vi "Log Event.vi"(0 "Robot Notifications in":refnum<class "Robot Event SystemLink.lvclass">, 1 "Program":string, 2 "data":variant, 5 "error in (no error)":errorcluster, 9 "Event Type":T1) -> (14 "Robot Notifications out":refnum<class "Robot Event SystemLink.lvclass">, 19 "error out":errorcluster)   [LabVIEW 2019, in "Robot Event SystemLink.lvclass"]
uses:
  Robot Event SystemLink.lvclass
  C:/_Code/Development/Sub-Zero Functional Test/standard hardware/Universal Robots/UR LabVIEW Interface/Classes/Events/Robot Event/Robot Event.lvclass
  Robot Event/Event Type.ctl
  Robot Event SystemLink.lvclass/Robot Event SystemLink.ctl
  <vilib>/Skyline/Alarm/Library/typedefs/Severity Level.ctl
  <vilib>/Skyline/Alarm/Library/typedefs/New Instance Information.ctl
  <vilib>/Skyline/Utilities/Property.ctl
  <vilib>/Skyline/Configuration/Configuration HTTP_class/NI Skyline Configuration HTTP.lvclass/NI Skyline Configuration HTTP.ctl
  <vilib>/Skyline/Notification/Class/NI SystemLink Notification.lvclass/NI SystemLink Notification.ctl
  <vilib>/Skyline/Notification/Class/Read Display Name.vi
  <vilib>/Skyline/Alarm/Class/Build Alarm Set Transition (Single Notification).vi
  <vilib>/Skyline/Configuration/Configuration HTTP_class/Read Configuration.vi
  <vilib>/Skyline/Notification/Class/Get Notification Strategies Core.vi
  <vilib>/Skyline/Notification/Class/Read ID.vi
  <vilib>/Skyline/Alarm/Class/Build Alarm Set Transition (Multiple Notifications).vi
  <vilib>/Skyline/Alarm/Class/Private/Add System to Properties.vi
  <vilib>/Skyline/Notification/Class/Initialize.vi
  <vilib>/Skyline/AssetManagement/Start Utilization (Single).vi
  <vilib>/Skyline/Utilities/Build Resource Name.vi
  <vilib>/Skyline/Utilities/Get Minion ID.vi
  <vilib>/Skyline/Utilities/Get System Name.vi
  <vilib>/Skyline/Alarm/Library/Community/Create or Update Alarm.vi
  <vilib>/Skyline/Configuration/Configuration HTTP_class/NI Skyline Configuration HTTP.lvclass
  <vilib>/Skyline/Notification/Class/NI SystemLink Notification.lvclass
  <vilib>/Skyline/Alarm/Class/NI SystemLink Alarm.lvclass
  <vilib>/Skyline/Alarm/Library/NI SystemLink Alarm Library.lvlib
  <vilib>/Skyline/Utilities/NI Skyline Utilities.lvlib
  <vilib>/Skyline/AssetManagement/NI SystemLink Asset Utilization.lvclass
  Robot Event/Robot Event.lvclass
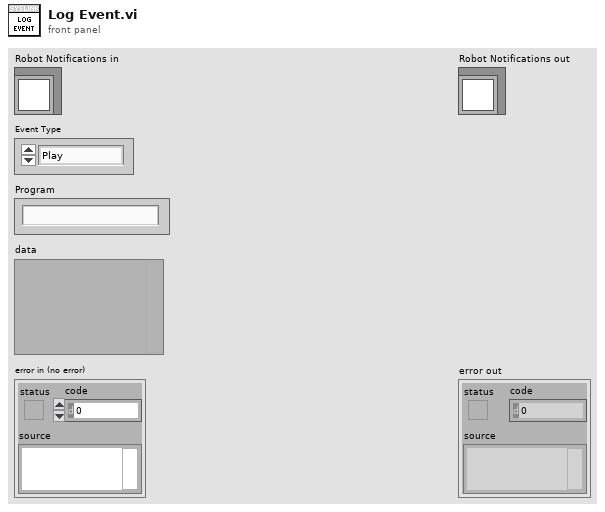
[diagram p1: front panel]
types:
  T1 = typedef "Robot Event.lvclass/Event Type.ctl" = enum16{"Play", "Error", "Fault", "Timeout", "Stopped", "Complete", "Fault - Program Resumed", "Fault - Program Aborted"}
  T2 = typedef "NI Skyline Utilities.lvlib/Property.ctl" = cluster{"key":string, "value":string}
  T3 = typedef "NI SystemLink Alarm Library.lvlib/New Instance Information.ctl" = cluster{"created by":string, "description":string, "keywords":string[], "properties":T2[]}
  T4 = typedef "NI SystemLink Alarm Library.lvlib/Severity Level.ctl" = i32
  T5 = typedef "NI SystemLink Alarm.lvclass/Set Transition.ctl" = cluster{"severity level":T4, "condition":string, "occurred at":timestamp, "notification strategies":refnum<class "NI SystemLink Notification.lvclass">[], "keywords":string[], "properties":T2[]}
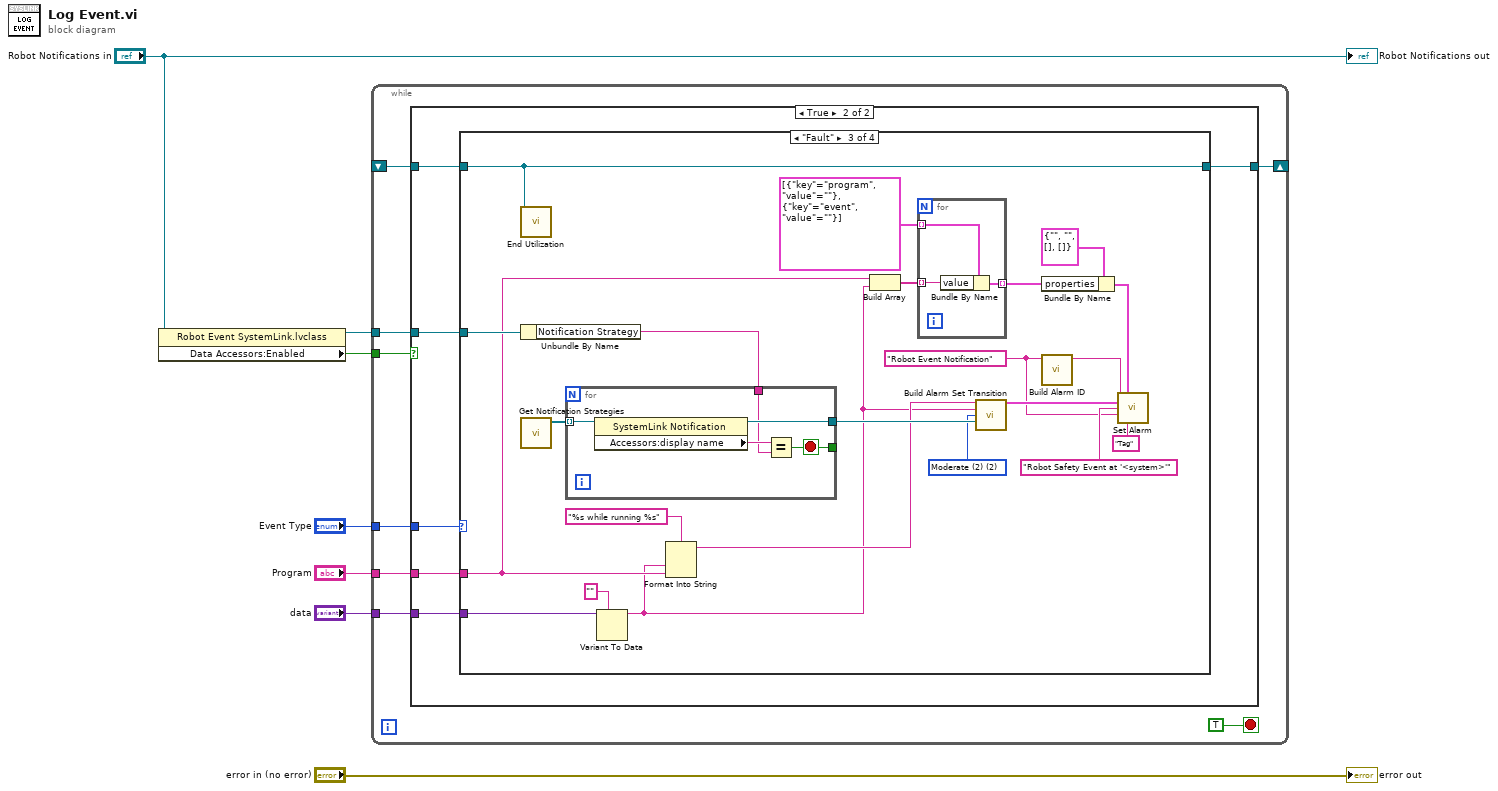
[diagram p0: block diagram]
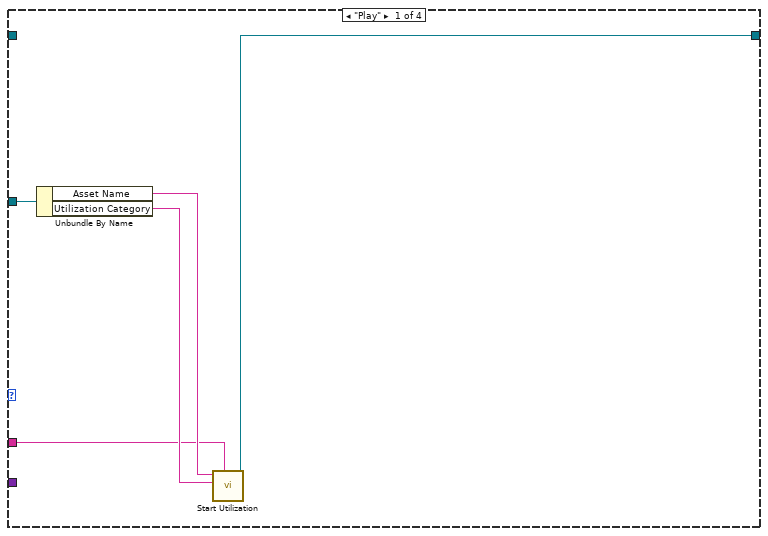
[diagram p3: hidden frame]
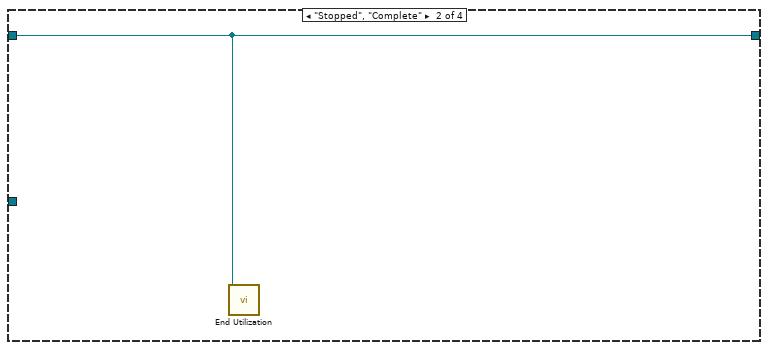
[diagram p4: hidden frame]
diagram:
  n1 = property class="Robot Event SystemLink.lvclass"(reference="Robot Notifications in") -> (reference out=w3:refnum<class "Robot Event SystemLink.lvclass">, "Data Accessors:Enabled"=w1:bool)  [unwired: 1 in, 1 out]
  n2 = while {
    tunnel: "Event Type" -> [w15]
    tunnel: "Program" -> [w14]
    tunnel: w3 -> [w13]
    tunnel: "data" -> [w12]
    tunnel: w1 -> [w11]
    shift-right: [w9] -> _
    shift-left: _ -> [w8]
    stop <- TRUE stop-if-true
    n3 = case shown="True" w11 {
      tunnel: w15 -> [_ w19]
      tunnel: w12 -> [_ w21]
      tunnel: w14 -> [_ w20]
      tunnel: w13 -> [_ w22]
      tunnel: [w16 w18] -> w9
      tunnel: w8 -> [w16 w17]
      frame False {
      }
      frame True {
        n4 = case shown="\"Fault\"" w19 {
          tunnel: w22 -> [w27 _ w50 _]
          tunnel: w21 -> [_ _ w45 _]
          tunnel: w20 -> [w23 _ w35 _]
          tunnel: [w24 w28 w29 w59] -> w18
          tunnel: w17 -> [_ w28 w29 w59]
          frame "Play" {
            n5 = Unbundle By Name(w27) -> ("Asset Name"=w26:string, "Utilization Category"=w25:string)
            n6 = call-poly <vilib>:"Start Utilization.vi"("task name"=w23, "utilization category"=w25, "asset name"=w26) -> ("asset utilization"=w24:refnum<class "NI SystemLink Asset Utilization.lvclass">)  [unwired: 7 in, 1 out]
          }
          frame "Stopped", "Complete" {
            n7 = call <vilib>:"End Utilization.vi"("asset utilization"=w28) -> ()  [unwired: 10 in, 1 out]
          }
          frame "Fault" {
            w38 = "Robot Event Notification" ("alarm name")
            w46 = T4 2 items=["Clear (-1)"=-1, "Low (1)"=1, "Moderate (2)"=2, "High (3)"=3, "Critical (4)"=4] ("severity level")
            n8 = call <vilib>:"End Utilization.vi"("asset utilization"=w29) -> ()  [unwired: 10 in, 1 out]
            n9 = Unbundle By Name(w50) -> ("Notification Strategy"=w48:string)
            n10 = call <vilib>:"Get Notification Strategies.vi"() -> ("notification strategies"=w49:refnum<class "NI SystemLink Notification.lvclass">[])  [unwired: 10 in, 1 out]
            n11 = for {
              tunnel: w49 -> [w58] mode=indexing
              tunnel: [w57] -> w47
              tunnel: w48 -> [w55]
              tunnel: [w54] -> _
              stop <- w54 stop-if-true
              n12 = property class="SystemLink Notification"(reference=w58) -> (reference out=w57:refnum<class "NI SystemLink Notification.lvclass">, "Accessors:display name"=w56:string)  [unwired: 1 in, 1 out]
              n13 = Equal?(x=w56, y=w55) -> (x = y?=w54:bool)
            }
            n14 = Variant To Data(type="", Variant=w45) -> (data=w34:string)  [unwired: 1 in, 1 out]
            n15 = Format Into String(format string="%s while running %s", w34, w35) -> (resulting string=w42:string)  [unwired: 2 in, 1 out]
            n16 = Build Array(w35, w34) -> (w33:string[])
            n17 = for {
              tunnel: w33 -> [w53] mode=indexing
              tunnel: [w52] -> w31 mode=indexing
              tunnel: T2[] [{"key"="program", "value"=""}, {"key"="event", "value"=""}] ("properties") -> [w51] mode=indexing
              n18 = Bundle By Name(cluster=w51, "value"=w53) -> (w52:T2)
            }
            n19 = call-poly <vilib>:"Build Alarm Set Transition.vi"("value"=w42, "condition"=w34, "severity level"=w46, "notification strategy"=w47) -> ("set transition"=w41:T5)  [unwired: 11 in]
            n20 = Bundle By Name(cluster=T3 {"created by"="", "description"="", "keywords"=[], "properties"=[]} ("additional information"), "properties"=w31) -> (w30:T3)
            n21 = call <vilib>:"Build Alarm ID.vi"("alarm name"=w38) -> ("alarm id"=w40:string)  [unwired: 10 in]
            n22 = call <vilib>:"Set Alarm.vi"("alarm id"=w40, "additional information"=w30, "set transition"=w41, "display name"="Robot Safety Event at '<system>'", "channel"=w38, "resource type"="Tag") -> ()  [unwired: 7 in, 3 out]
          }
          frame Default {
          }
        }
      }
    }
  }
  "error out" <- "error in (no error)"
  "Robot Notifications out" <- "Robot Notifications in"
